vi "Run.vi"(8 "error in (no error)":errorcluster, 11 "LUnit Test Suite In":refnum<class "LUnit Test Suite.lvclass">) -> (0 "error out":errorcluster, 1 "Done?":bool, 2 "Results":T1[](array[typedef]), 3 "LUnit Test Suite In 2":refnum<class "LUnit Test Suite.lvclass">)   [LabVIEW 2020, in "LUnit Test Suite.lvclass"]
doc: "Execute next test in suite. Done indicator is True if the test suite is exhausted and all active tests have been run."
uses:
  LUnit Test Suite.lvclass
  Result/Result.ctl
  Result/Status.ctl
  Result/Type.ctl
  LUnit Test Suite.lvclass/LUnit Test Suite.ctl
  <vilib>/Utility/miscctls.llb/LVMapReplaceAction.ctl
  Runnable/Runnable.lvclass
  Result/Result.lvlib
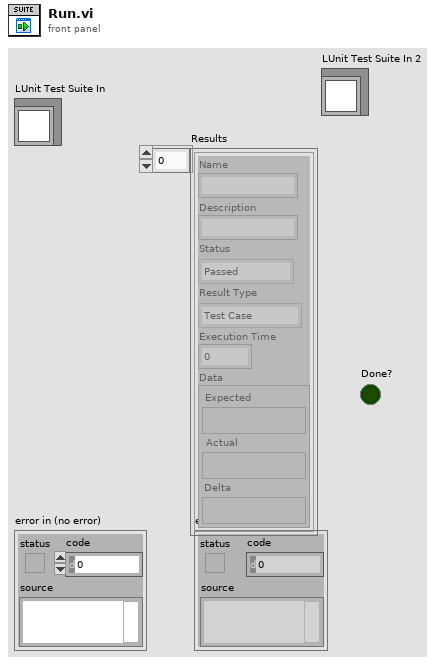
[diagram p1: front panel]
types:
  T1 = typedef "Result.lvlib/Result.ctl" = cluster{"Name":string, "Description":string, "Status":T2, "Result Type":T3, "Execution Time":dbl, "Data":cluster{"Expected":variant, "Actual":variant, "Delta":variant}}
  T2 = typedef "Result.lvlib/Status.ctl" = enum16{"", "Passed", "Failed", "Error", "Skipped", "Setup Error", "Broken", "Teardown Error"}
  T3 = typedef "Result.lvlib/Type.ctl" = enum16{"Test Case", "Test Suite", "Test Run", "Pass", "Fail", "Skip", "Pass if", "Fail if", "Pass if Error", "Fail if Error", "Pass if Equal", "Fail if Equal"}
  T4 = typedef "LVMapReplaceAction.ctl" = enum32{"Modify Entry only if found", "Add or Modify Entry", "Delete Entry"}
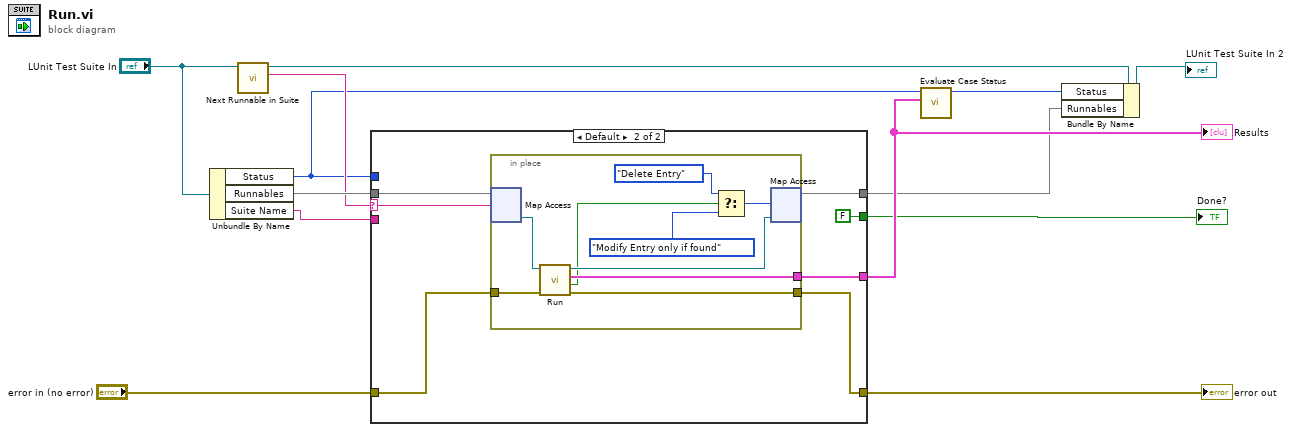
[diagram p0: block diagram]
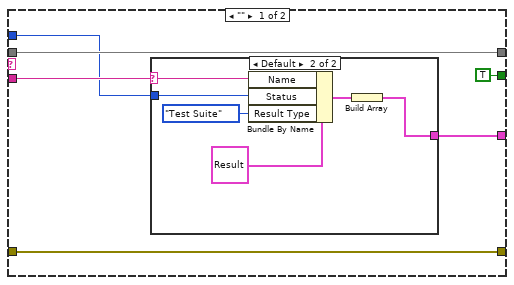
[diagram p2: hidden frame]
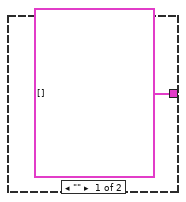
[diagram p3: hidden frame]
diagram:
  n1 = Unbundle By Name("LUnit Test Suite In") -> ("Status"=w1:T2, "Runnables"=w7:map{string, refnum<class "Runnable.lvclass">}, "Suite Name"=w2:string)
  n2 = call "Next Runnable in Suite.vi"("LUnit Test Suite In"="LUnit Test Suite In") -> ("Next"=w5:string, "LUnit Test Suite Out"=w4:refnum<class "LUnit Test Suite.lvclass">)  [unwired: 8 in, 1 out]
  n3 = case shown="Default" w5 {
    selector: w5 -> [_ w27]
    tunnel: "error in (no error)" -> [w17 w33]
    tunnel: [w17 w32] -> w12
    tunnel: w7 -> [w19 w28]
    tunnel: [w18 w31] -> w9
    tunnel: [w19 w30] -> w8
    tunnel: [TRUE FALSE] -> w6
    tunnel: w2 -> [w15 _]
    tunnel: w1 -> [w14 _]
    frame "" {
      n4 = case shown="Default" w15 {
        selector: w15 -> [_ w25]
        tunnel: w14 -> [_ w24]
        tunnel: [T1[] [] w22] -> w18
        frame "" {
        }
        frame Default {
          n5 = Bundle By Name(cluster=T1 {"Name"="", "Description"="", "Status"=enum."Passed", "Result Type"=enum."Test Case", "Execution Time"=0.0, "Data"={"Expected"=variant, "Actual"=variant, "Delta"=variant}} ("Results"), "Name"=w25, "Status"=w24, "Result Type"=Type."Test Suite") -> (w23:T1)
          n6 = Build Array(w23) -> (w22:T1[])
        }
      }
    }
    frame Default {
      n7 = in-place {
        in-place-border: w33 -> [w42]
        in-place-border: [w41] -> w32
        in-place-border: [w40] -> w31
        n8 = in-place-map #1(w28, w27) -> (w38:refnum<class "Runnable.lvclass">)  [unwired: 1 in, 1 out]
        n9 = call-dynamic "Run.vi"("error in (no error)"=w42, "Runnable In"=w38) -> ("error out"=w41:errorcluster, "Done?"=w37:bool, "Results"=w40:T1[], "Runnable Out"=w39:refnum<class "Runnable.lvclass">)  [unwired: 6 in]
        n10 = Select(t=LVMapReplaceAction."Delete Entry" ("action"), s=w37, f=LVMapReplaceAction."Modify Entry only if found" ("action")) -> (s? t:f=w34:T4)
        n11 = in-place-map #1(w39, w34) -> (w30:map{string, refnum<class "Runnable.lvclass">})  [unwired: 2 out]
      }
    }
  }
  "error out" <- w12
  "Results" <- w9
  "Done?" <- w6
  n12 = call "Evaluate Case Status.vi"("Results"=w9, "Current"=w1) -> ("Status"=w10:T2)  [unwired: 9 in]
  n13 = Bundle By Name(cluster=w4, "Status"=w10, "Runnables"=w8) -> (→"LUnit Test Suite In 2":refnum<class "LUnit Test Suite.lvclass">)
